vi "Down Pressure.vi"(5 "Direction":T1, 7 "init":bool, 8 "error in (no error)":errorcluster, 11 "Stand in":refnum<class "Stand.lvclass">) -> (0 "error out":errorcluster, 2 "done":bool, 3 "Stand out":refnum<class "Stand.lvclass">)   [LabVIEW 2019, in "Stand.lvclass"]
uses:
  Stand.lvclass
  TypeDef/Direction.ctl
  C:/Users/ANENKOV_V1/Desktop/src/Device_class/Device.lvclass
  TypeDef/State - Pressure Down.ctl
  Stand.lvclass/Stand.ctl
  AI_class/AI.lvclass/AI.ctl
  AnalogComparator_class/AnalogComparator.lvclass/AnalogComparator.ctl
  Device_class/Device.lvclass/Device.ctl
  FPGA/TypeDef/DO index.ctl
  NeedleValve_class/Cmd.ctl
  f8234472-8bf1-448c-8c25-8d9f60be58e1.vi
  AnalogComparator_class/GetStatus.vi
  FPGA_API_class/FPGA API.lvclass
  Device_class/Device.lvclass
  AI_class/AI.lvclass
  NeedleValve_class/NeedleValve.lvclass
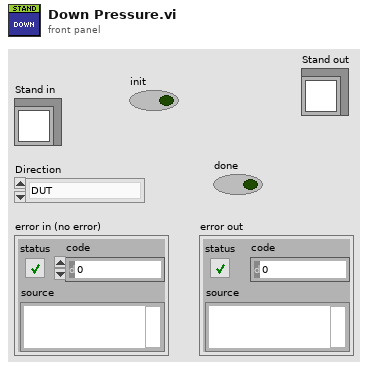
[diagram p1: front panel]
types:
  T1 = typedef "Direction.ctl" = enum8{"DUT", "Chamber"}
  T2 = typedef "State - Pressure Down.ctl" = enum16{"Check", "Close Inlet", "Open Outlet", "Down", "Exit"}
  T3 = typedef "NeedleValve.lvclass/Cmd.ctl" = enum16{"Open", "Close", "Stop"}
  T4 = typedef "AI_Data.ctl" = cluster{"Stat Data":T5, "OutOfRangeMax":bool, "OutOfRangeMin":bool, "HIHI":bool, "HI":bool, "LO":bool, "LOLO":bool}
  T5 = typedef "AI Statistics Data.ctl" = cluster{"raw mean":dbl, "scl mean":dbl, "raw mean 1Hz":dbl, "scl mean 1Hz":dbl}
  T6 = typedef "DO index.ctl" = u8
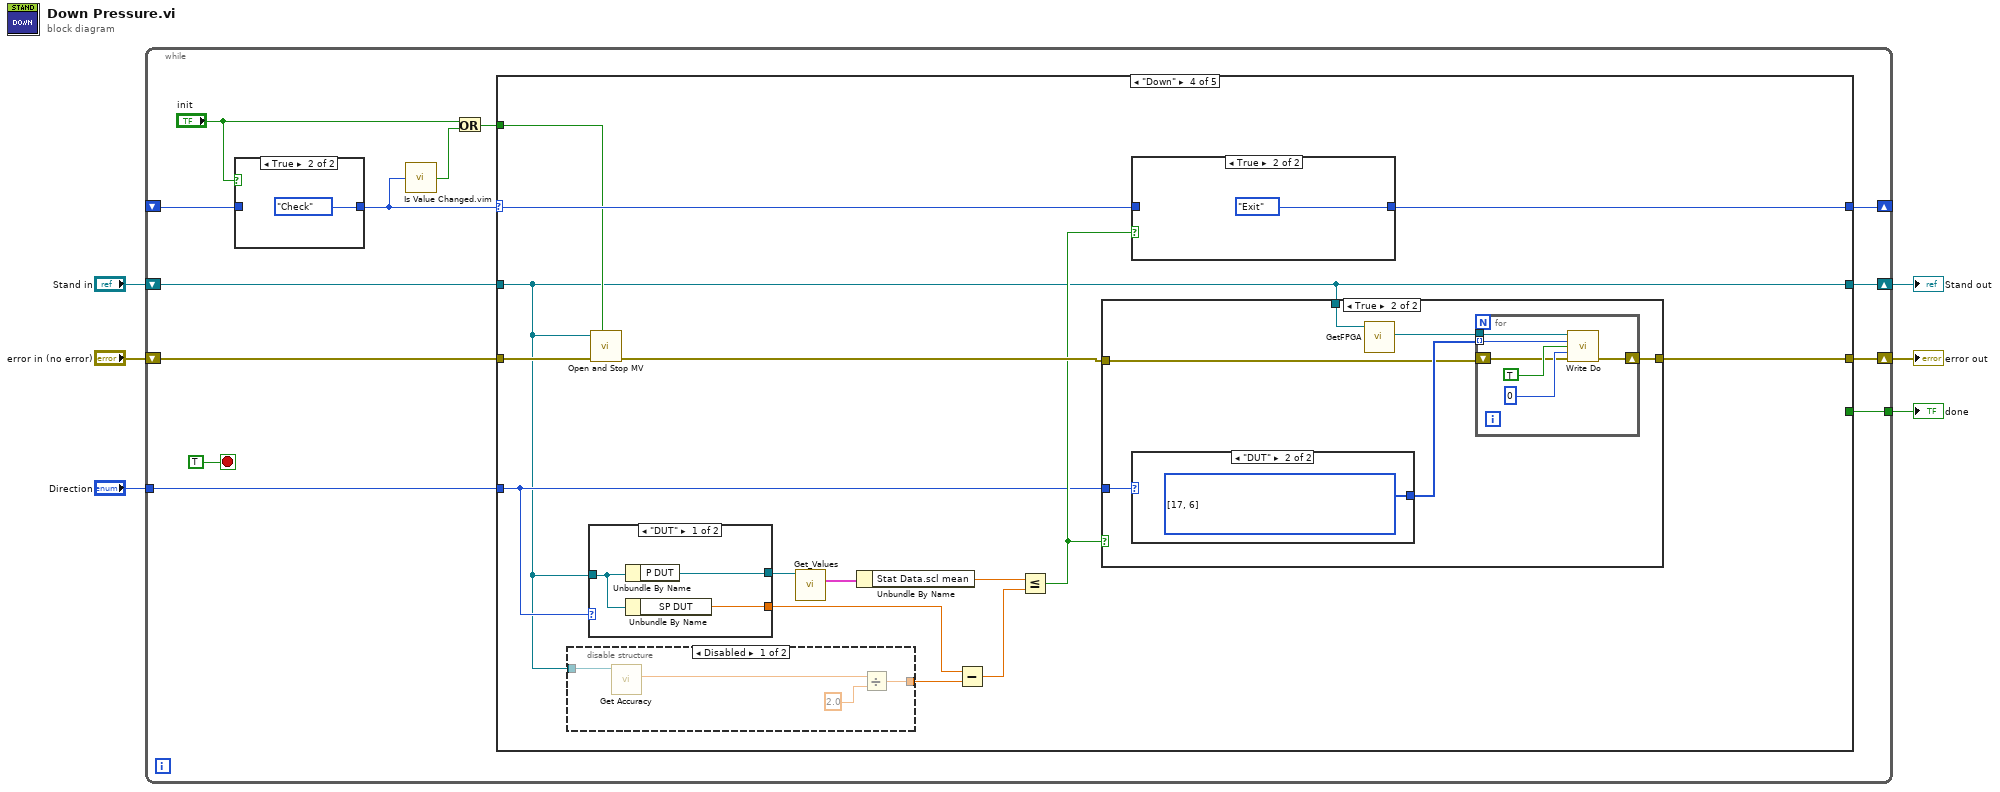
[diagram p0: block diagram]
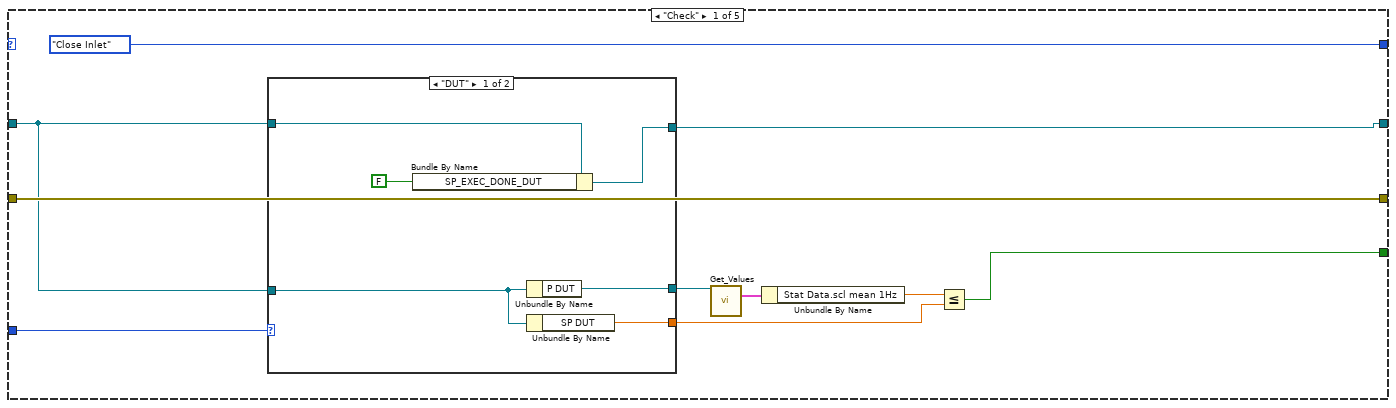
[diagram p2: hidden frame]
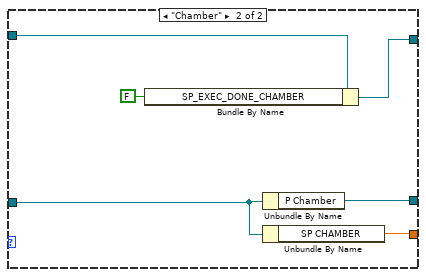
[diagram p3: hidden frame]
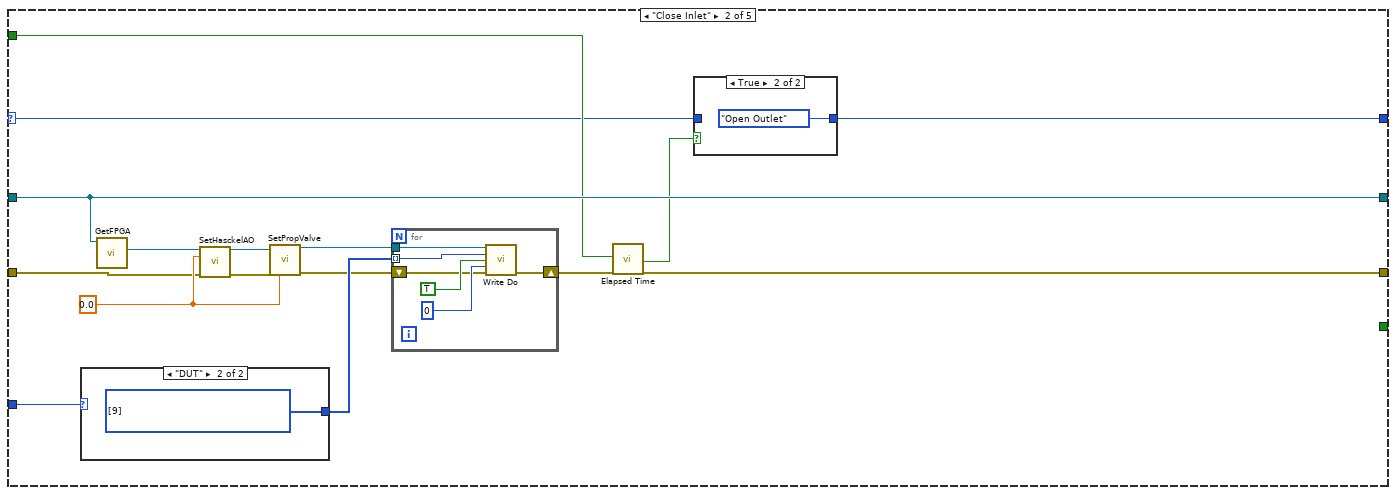
[diagram p4: hidden frame]
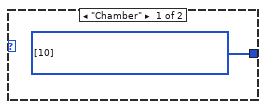
[diagram p6: hidden frame]
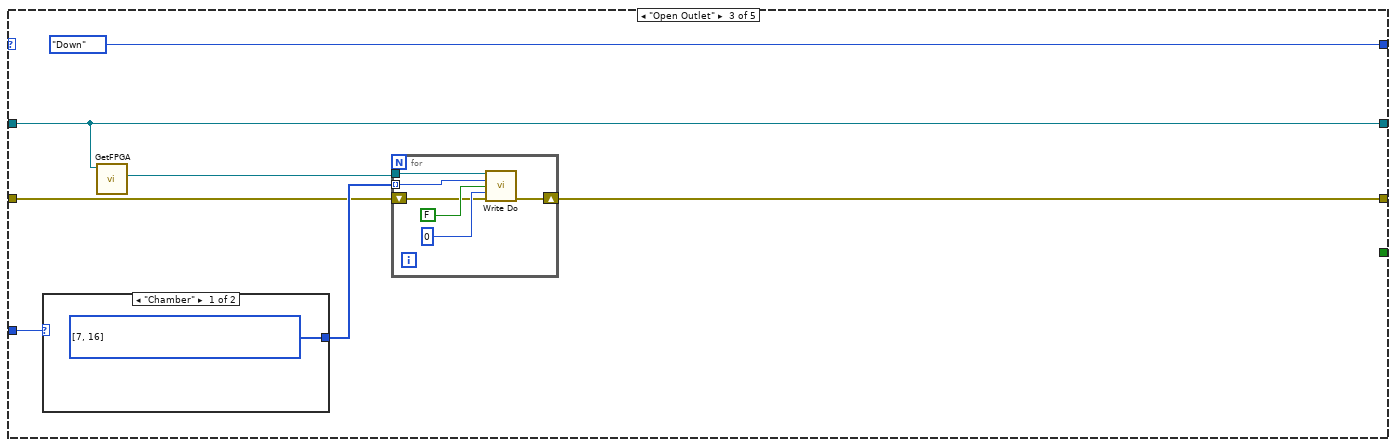
[diagram p7: hidden frame]
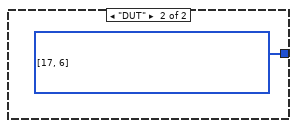
[diagram p8: hidden frame]
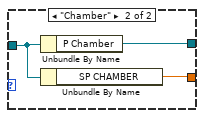
[diagram p10: hidden frame]
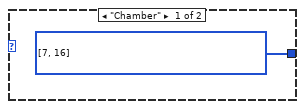
[diagram p13: hidden frame]
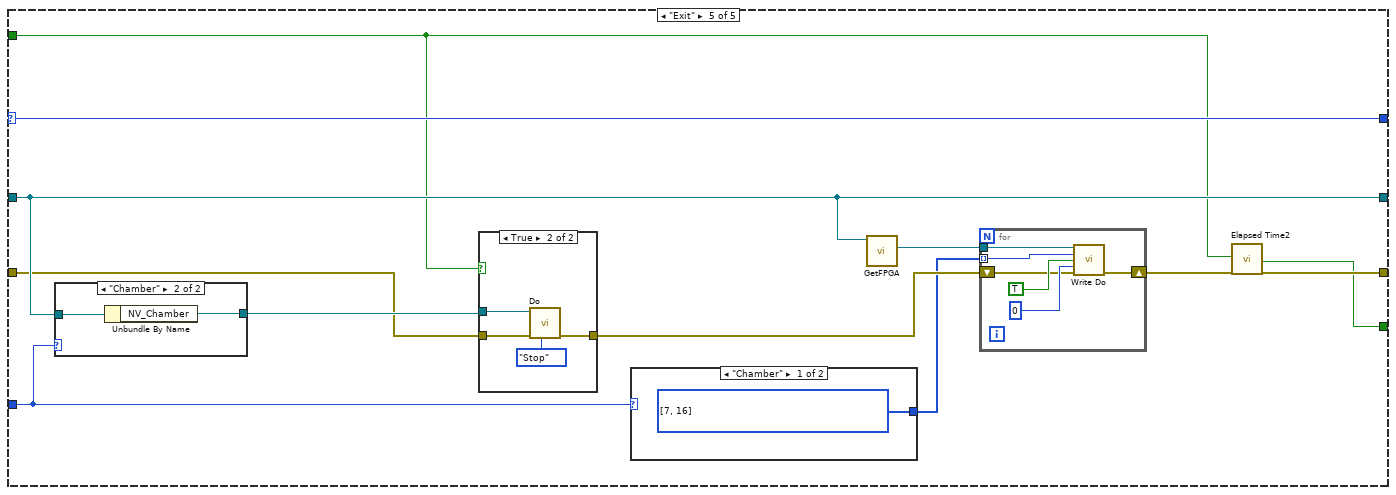
[diagram p14: hidden frame]
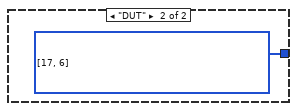
[diagram p15: hidden frame]
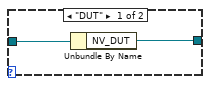
[diagram p17: hidden frame]
diagram:
  n1 = while {
    shift-right: [w11] -> w2
    shift-left: "error in (no error)" -> [w10]
    tunnel: "Direction" -> [w7]
    shift-right: [w12] -> w3
    shift-left: "Stand in" -> [w9]
    shift-right: [w18] -> _
    shift-left: _ -> [w17]
    tunnel: [w8] -> w1
    stop <- TRUE stop-if-true
    n2 = case shown="True" "init" {
      tunnel: [w154 State_-_Pressure_Down."Check"] -> w16
      tunnel: w17 -> [w154 _]
      frame False {
      }
      frame True {
      }
    }
    n3 = call "Is Value Changed.vim"("value"=w16) -> ("changed or first call?"=w14:bool)
    n4 = Or(x="init", y=w14) -> (x .or. y?=w13:bool)
    n5 = case shown="\"Down\"" w16 {
      selector: w16 -> [_ w44 _ w93 w133]
      tunnel: w9 -> [w21 w49 w71 w86 w135]
      tunnel: [State_-_Pressure_Down."Close Inlet" w45 State_-_Pressure_Down."Down" w94 w133] -> w18
      tunnel: w13 -> [_ w47 _ w87 w126]
      tunnel: [w20 w49 w71 w86 w135] -> w12
      tunnel: [w29 w43 w70 w97 w127] -> w11
      tunnel: w10 -> [w29 w50 w72 w95 w129]
      tunnel: w7 -> [w23 w42 w68 w88 w136]
      tunnel: [w22 _ _ _ w125] -> w8
      frame "Check" {
        n6 = case shown="\"DUT\"" w23 {
          tunnel: [w35 w41] -> w26
          tunnel: [w34 w40] -> w24
          tunnel: w21 -> [w33 w39]
          tunnel: w21 -> [w31 w38]
          tunnel: [w30 w37] -> w20
          frame "DUT" {
            n7 = Bundle By Name(cluster=w31, "SP_EXEC_DONE_DUT"=FALSE ("Data.STS.SP_EXEC_DONE_CHAMBER")) -> (w30:refnum<class "Stand.lvclass">)
            n8 = Unbundle By Name(w33) -> ("P DUT"=w35:refnum<class "AI.lvclass">)
            n9 = Unbundle By Name(w33) -> ("SP DUT"=w34:dbl)
          }
          frame "Chamber" {
            n10 = Bundle By Name(cluster=w38, "SP_EXEC_DONE_CHAMBER"=FALSE ("Data.STS.SP_EXEC_DONE_CHAMBER")) -> (w37:refnum<class "Stand.lvclass">)
            n11 = Unbundle By Name(w39) -> ("P Chamber"=w41:refnum<class "AI.lvclass">)
            n12 = Unbundle By Name(w39) -> ("SP CHAMBER"=w40:dbl)
          }
        }
        n13 = call "Get_Values.vi"("reference in"=w26) -> ("Data"=w27:T4)  [unwired: 14 in]
        n14 = Unbundle By Name(w27) -> ("Stat Data.scl mean 1Hz"=w25:dbl)
        n15 = Less Or Equal?(x=w25, y=w24) -> (x <= y?=w22:bool)
      }
      frame "Close Inlet" {
        w51 = 0.0 ("Haskel in")
        n16 = case shown="\"DUT\"" w42 {
          tunnel: [w66 w67] -> w57
          frame "Chamber" {
            w66 = T6[] [10] items=["DO 0 [KP1] [M12]", "DO 1 [ON KP2] [M21]", "DO 2 [ON KP3] [M24]", "DO 3 [WATER Y18.1 [DO3]]", "DO 4 [WATER Y18.2 [DO4]]", "DO 5 [KP6 Y29.1 33.7]", "DO 6 [KP7 Y29.2 33.8]", "DO 7 [KP8 Y29.3 33.9]", "DO 8 [KP9 Y29.4  33.12]", "DO 9 [KP10 Y29.5 33.1]", "DO 10 [KP11 Y29.6 33.2]", "DO 11 [KP12 Y29.7  33.13]", "DO 12 [KP13 Y29.8  33.11]", "DO 13 [KP14 Y29.9 33.10]", "DO 14 [KP15 Y29.10  33.6]", "DO 15 [KP16 Y29.11  33.5]", "DO 16 [KP17 Y29.12  33.4]", "DO 17 [KP18 Y29.13 33.3]", "DO 18 [AIR KP19]", "DO 19 [STEP DRIVE EN KP20]", "DO 20 [KP21 Y44.1 OPEN]", "DO 21 [ KP22 Y44.1 CLOSE]", "DO 22 [ KP23 Y44.2 OPEN]", "DO 23", "DO 24 [STEP DRIVE 1]", "DO 25 [STEP DRIVE 2]"]
          }
          frame "DUT" {
            w67 = T6[] [9] items=["DO 0 [KP1] [M12]", "DO 1 [ON KP2] [M21]", "DO 2 [ON KP3] [M24]", "DO 3 [WATER Y18.1 [DO3]]", "DO 4 [WATER Y18.2 [DO4]]", "DO 5 [KP6 Y29.1 33.7]", "DO 6 [KP7 Y29.2 33.8]", "DO 7 [KP8 Y29.3 33.9]", "DO 8 [KP9 Y29.4  33.12]", "DO 9 [KP10 Y29.5 33.1]", "DO 10 [KP11 Y29.6 33.2]", "DO 11 [KP12 Y29.7  33.13]", "DO 12 [KP13 Y29.8  33.11]", "DO 13 [KP14 Y29.9 33.10]", "DO 14 [KP15 Y29.10  33.6]", "DO 15 [KP16 Y29.11  33.5]", "DO 16 [KP17 Y29.12  33.4]", "DO 17 [KP18 Y29.13 33.3]", "DO 18 [AIR KP19]", "DO 19 [STEP DRIVE EN KP20]", "DO 20 [KP21 Y44.1 OPEN]", "DO 21 [ KP22 Y44.1 CLOSE]", "DO 22 [ KP23 Y44.2 OPEN]", "DO 23", "DO 24 [STEP DRIVE 1]", "DO 25 [STEP DRIVE 2]"]
          }
        }
        n17 = call "GetFPGA.vi"("Device in"=w49) -> ("FPGA API.lvclass"=w52:refnum<class "FPGA API.lvclass">)  [unwired: 10 in]
        n18 = call-dynamic "SetHasckelAO.vi"("FPGA API in"=w52, "Haskel in"=w51, "error in (no error)"=w50) -> ("FPGA API out"=w54:refnum<class "FPGA API.lvclass">, "error out"=w53:errorcluster)  [unwired: 11 in]
        n19 = call-dynamic "SetPropValve.vi"("FPGA API in"=w54, "error in (no error)"=w53, "AO 1"=w51) -> ("FPGA API out"=w55:refnum<class "FPGA API.lvclass">, "error out"=w56:errorcluster)  [unwired: 11 in]
        n20 = for {
          tunnel: w55 -> [w63]
          tunnel: w57 -> [w61] mode=indexing
          shift-right: [w60] -> w48
          shift-left: w56 -> [w62]
          n21 = call-dynamic "Write Do.vi"("FPGA API in"=w63, "#DO"=w61, "value"=TRUE, "Time uSec"=u32 0, "error in (no error)"=w62) -> ("error out"=w60:errorcluster)  [unwired: 9 in, 1 out]
        }
        n22 = call "Elapsed Time"("Reset"=w47, "error in (no error)"=w48) -> ("Time has Elapsed"=w46:bool, "error out"=w43:errorcluster)  [unwired: 10 in, 6 out]
        n23 = case shown="True" w46 {
          tunnel: [w58 State_-_Pressure_Down."Open Outlet"] -> w45
          tunnel: w44 -> [w58 _]
          frame False {
          }
          frame True {
          }
        }
      }
      frame "Open Outlet" {
        n24 = case shown="\"Chamber\"" w68 {
          tunnel: [w81 w82] -> w74
          frame "Chamber" {
            w81 = T6[] [7, 16] items=["DO 0 [KP1] [M12]", "DO 1 [ON KP2] [M21]", "DO 2 [ON KP3] [M24]", "DO 3 [WATER Y18.1 [DO3]]", "DO 4 [WATER Y18.2 [DO4]]", "DO 5 [KP6 Y29.1 33.7]", "DO 6 [KP7 Y29.2 33.8]", "DO 7 [KP8 Y29.3 33.9]", "DO 8 [KP9 Y29.4  33.12]", "DO 9 [KP10 Y29.5 33.1]", "DO 10 [KP11 Y29.6 33.2]", "DO 11 [KP12 Y29.7  33.13]", "DO 12 [KP13 Y29.8  33.11]", "DO 13 [KP14 Y29.9 33.10]", "DO 14 [KP15 Y29.10  33.6]", "DO 15 [KP16 Y29.11  33.5]", "DO 16 [KP17 Y29.12  33.4]", "DO 17 [KP18 Y29.13 33.3]", "DO 18 [AIR KP19]", "DO 19 [STEP DRIVE EN KP20]", "DO 20 [KP21 Y44.1 OPEN]", "DO 21 [ KP22 Y44.1 CLOSE]", "DO 22 [ KP23 Y44.2 OPEN]", "DO 23", "DO 24 [STEP DRIVE 1]", "DO 25 [STEP DRIVE 2]"]
          }
          frame "DUT" {
            w82 = T6[] [17, 6] items=["DO 0 [KP1] [M12]", "DO 1 [ON KP2] [M21]", "DO 2 [ON KP3] [M24]", "DO 3 [WATER Y18.1 [DO3]]", "DO 4 [WATER Y18.2 [DO4]]", "DO 5 [KP6 Y29.1 33.7]", "DO 6 [KP7 Y29.2 33.8]", "DO 7 [KP8 Y29.3 33.9]", "DO 8 [KP9 Y29.4  33.12]", "DO 9 [KP10 Y29.5 33.1]", "DO 10 [KP11 Y29.6 33.2]", "DO 11 [KP12 Y29.7  33.13]", "DO 12 [KP13 Y29.8  33.11]", "DO 13 [KP14 Y29.9 33.10]", "DO 14 [KP15 Y29.10  33.6]", "DO 15 [KP16 Y29.11  33.5]", "DO 16 [KP17 Y29.12  33.4]", "DO 17 [KP18 Y29.13 33.3]", "DO 18 [AIR KP19]", "DO 19 [STEP DRIVE EN KP20]", "DO 20 [KP21 Y44.1 OPEN]", "DO 21 [ KP22 Y44.1 CLOSE]", "DO 22 [ KP23 Y44.2 OPEN]", "DO 23", "DO 24 [STEP DRIVE 1]", "DO 25 [STEP DRIVE 2]"]
          }
        }
        n25 = call "GetFPGA.vi"("Device in"=w71) -> ("FPGA API.lvclass"=w73:refnum<class "FPGA API.lvclass">)  [unwired: 10 in]
        n26 = for {
          tunnel: w73 -> [w78]
          tunnel: w74 -> [w76] mode=indexing
          shift-right: [w75] -> w70
          shift-left: w72 -> [w77]
          n27 = call-dynamic "Write Do.vi"("FPGA API in"=w78, "#DO"=w76, "value"=FALSE, "Time uSec"=u32 0, "error in (no error)"=w77) -> ("error out"=w75:errorcluster)  [unwired: 9 in, 1 out]
        }
      }
      frame "Down" {
        n28 = disable-structure shown="Disabled" {
          disable-tunnel: w86 -> [w100 _]
          disable-tunnel: [w98 _] -> w85
          frame Disabled {
            n29 = call "Get Accuracy.vi"("Stand in"=w100) -> ("Accuracy [MPa]"=w99:dbl)  [unwired: 10 in]
            n30 = Divide(x=w99, y=2.0) -> (x/y=w98:dbl)
          }
          frame Enabled {
          }
        }
        n31 = case shown="\"DUT\"" w88 {
          tunnel: [w104 w107] -> w91
          tunnel: [w103 w106] -> w84
          tunnel: w86 -> [w102 w105]
          frame "DUT" {
            n32 = Unbundle By Name(w102) -> ("P DUT"=w104:refnum<class "AI.lvclass">)
            n33 = Unbundle By Name(w102) -> ("SP DUT"=w103:dbl)
          }
          frame "Chamber" {
            n34 = Unbundle By Name(w105) -> ("P Chamber"=w107:refnum<class "AI.lvclass">)
            n35 = Unbundle By Name(w105) -> ("SP CHAMBER"=w106:dbl)
          }
        }
        n36 = call "Open and Stop MV.vi"("init"=w87, "error in (no error)"=w95, "Stand in"=w86) -> ("error out"=w96:errorcluster)  [unwired: 8 in]
        n37 = call "Get_Values.vi"("reference in"=w91) -> ("Data"=w92:T4)  [unwired: 14 in]
        n38 = Unbundle By Name(w92) -> ("Stat Data.scl mean"=w90:dbl)
        n39 = Subtract(x=w84, y=w85) -> (x-y=w83:dbl)
        n40 = Less Or Equal?(x=w90, y=w83) -> (x <= y?=w89:bool)
        n41 = case shown="True" w89 {
          tunnel: w88 -> [_ w114]
          tunnel: [w110 w113] -> w97
          tunnel: w86 -> [_ w112]
          tunnel: w96 -> [w110 w111]
          frame False {
          }
          frame True {
            n42 = case shown="\"DUT\"" w114 {
              tunnel: [w123 w124] -> w116
              frame "Chamber" {
                w123 = T6[] [7, 16] items=["DO 0 [KP1] [M12]", "DO 1 [ON KP2] [M21]", "DO 2 [ON KP3] [M24]", "DO 3 [WATER Y18.1 [DO3]]", "DO 4 [WATER Y18.2 [DO4]]", "DO 5 [KP6 Y29.1 33.7]", "DO 6 [KP7 Y29.2 33.8]", "DO 7 [KP8 Y29.3 33.9]", "DO 8 [KP9 Y29.4  33.12]", "DO 9 [KP10 Y29.5 33.1]", "DO 10 [KP11 Y29.6 33.2]", "DO 11 [KP12 Y29.7  33.13]", "DO 12 [KP13 Y29.8  33.11]", "DO 13 [KP14 Y29.9 33.10]", "DO 14 [KP15 Y29.10  33.6]", "DO 15 [KP16 Y29.11  33.5]", "DO 16 [KP17 Y29.12  33.4]", "DO 17 [KP18 Y29.13 33.3]", "DO 18 [AIR KP19]", "DO 19 [STEP DRIVE EN KP20]", "DO 20 [KP21 Y44.1 OPEN]", "DO 21 [ KP22 Y44.1 CLOSE]", "DO 22 [ KP23 Y44.2 OPEN]", "DO 23", "DO 24 [STEP DRIVE 1]", "DO 25 [STEP DRIVE 2]"]
              }
              frame "DUT" {
                w124 = T6[] [17, 6] items=["DO 0 [KP1] [M12]", "DO 1 [ON KP2] [M21]", "DO 2 [ON KP3] [M24]", "DO 3 [WATER Y18.1 [DO3]]", "DO 4 [WATER Y18.2 [DO4]]", "DO 5 [KP6 Y29.1 33.7]", "DO 6 [KP7 Y29.2 33.8]", "DO 7 [KP8 Y29.3 33.9]", "DO 8 [KP9 Y29.4  33.12]", "DO 9 [KP10 Y29.5 33.1]", "DO 10 [KP11 Y29.6 33.2]", "DO 11 [KP12 Y29.7  33.13]", "DO 12 [KP13 Y29.8  33.11]", "DO 13 [KP14 Y29.9 33.10]", "DO 14 [KP15 Y29.10  33.6]", "DO 15 [KP16 Y29.11  33.5]", "DO 16 [KP17 Y29.12  33.4]", "DO 17 [KP18 Y29.13 33.3]", "DO 18 [AIR KP19]", "DO 19 [STEP DRIVE EN KP20]", "DO 20 [KP21 Y44.1 OPEN]", "DO 21 [ KP22 Y44.1 CLOSE]", "DO 22 [ KP23 Y44.2 OPEN]", "DO 23", "DO 24 [STEP DRIVE 1]", "DO 25 [STEP DRIVE 2]"]
              }
            }
            n43 = call "GetFPGA.vi"("Device in"=w112) -> ("FPGA API.lvclass"=w115:refnum<class "FPGA API.lvclass">)  [unwired: 10 in]
            n44 = for {
              tunnel: w115 -> [w120]
              tunnel: w116 -> [w118] mode=indexing
              shift-right: [w117] -> w113
              shift-left: w111 -> [w119]
              n45 = call-dynamic "Write Do.vi"("FPGA API in"=w120, "#DO"=w118, "value"=TRUE, "Time uSec"=u32 0, "error in (no error)"=w119) -> ("error out"=w117:errorcluster)  [unwired: 9 in, 1 out]
            }
          }
        }
        n46 = case shown="True" w89 {
          tunnel: [w108 State_-_Pressure_Down."Exit"] -> w94
          tunnel: w93 -> [w108 _]
          frame False {
          }
          frame True {
          }
        }
      }
      frame "Exit" {
        n47 = case shown="\"Chamber\"" w136 {
          tunnel: [w151 w153] -> w130
          tunnel: w135 -> [w150 w152]
          frame "DUT" {
            n48 = Unbundle By Name(w150) -> ("NV_DUT"=w151:refnum<class "NeedleValve.lvclass">)
          }
          frame "Chamber" {
            n49 = Unbundle By Name(w152) -> ("NV_Chamber"=w153:refnum<class "NeedleValve.lvclass">)
          }
        }
        n50 = case shown="True" w126 {
          tunnel: [w145 w149] -> w134
          tunnel: w130 -> [_ w147]
          tunnel: w129 -> [w145 w146]
          frame False {
          }
          frame True {
            n51 = call "Do.vi"("Cmd"=Cmd."Stop", "error in (no error)"=w146, "NeedleValve in"=w147) -> ("error out"=w149:errorcluster)  [unwired: 7 in, 1 out]
          }
        }
        n52 = case shown="\"Chamber\"" w136 {
          tunnel: [w143 w144] -> w132
          frame "Chamber" {
            w143 = T6[] [7, 16] items=["DO 0 [KP1] [M12]", "DO 1 [ON KP2] [M21]", "DO 2 [ON KP3] [M24]", "DO 3 [WATER Y18.1 [DO3]]", "DO 4 [WATER Y18.2 [DO4]]", "DO 5 [KP6 Y29.1 33.7]", "DO 6 [KP7 Y29.2 33.8]", "DO 7 [KP8 Y29.3 33.9]", "DO 8 [KP9 Y29.4  33.12]", "DO 9 [KP10 Y29.5 33.1]", "DO 10 [KP11 Y29.6 33.2]", "DO 11 [KP12 Y29.7  33.13]", "DO 12 [KP13 Y29.8  33.11]", "DO 13 [KP14 Y29.9 33.10]", "DO 14 [KP15 Y29.10  33.6]", "DO 15 [KP16 Y29.11  33.5]", "DO 16 [KP17 Y29.12  33.4]", "DO 17 [KP18 Y29.13 33.3]", "DO 18 [AIR KP19]", "DO 19 [STEP DRIVE EN KP20]", "DO 20 [KP21 Y44.1 OPEN]", "DO 21 [ KP22 Y44.1 CLOSE]", "DO 22 [ KP23 Y44.2 OPEN]", "DO 23", "DO 24 [STEP DRIVE 1]", "DO 25 [STEP DRIVE 2]"]
          }
          frame "DUT" {
            w144 = T6[] [17, 6] items=["DO 0 [KP1] [M12]", "DO 1 [ON KP2] [M21]", "DO 2 [ON KP3] [M24]", "DO 3 [WATER Y18.1 [DO3]]", "DO 4 [WATER Y18.2 [DO4]]", "DO 5 [KP6 Y29.1 33.7]", "DO 6 [KP7 Y29.2 33.8]", "DO 7 [KP8 Y29.3 33.9]", "DO 8 [KP9 Y29.4  33.12]", "DO 9 [KP10 Y29.5 33.1]", "DO 10 [KP11 Y29.6 33.2]", "DO 11 [KP12 Y29.7  33.13]", "DO 12 [KP13 Y29.8  33.11]", "DO 13 [KP14 Y29.9 33.10]", "DO 14 [KP15 Y29.10  33.6]", "DO 15 [KP16 Y29.11  33.5]", "DO 16 [KP17 Y29.12  33.4]", "DO 17 [KP18 Y29.13 33.3]", "DO 18 [AIR KP19]", "DO 19 [STEP DRIVE EN KP20]", "DO 20 [KP21 Y44.1 OPEN]", "DO 21 [ KP22 Y44.1 CLOSE]", "DO 22 [ KP23 Y44.2 OPEN]", "DO 23", "DO 24 [STEP DRIVE 1]", "DO 25 [STEP DRIVE 2]"]
          }
        }
        n53 = call "GetFPGA.vi"("Device in"=w135) -> ("FPGA API.lvclass"=w131:refnum<class "FPGA API.lvclass">)  [unwired: 10 in]
        n54 = for {
          tunnel: w131 -> [w140]
          tunnel: w132 -> [w138] mode=indexing
          shift-right: [w137] -> w128
          shift-left: w134 -> [w139]
          n55 = call-dynamic "Write Do.vi"("FPGA API in"=w140, "#DO"=w138, "value"=TRUE, "Time uSec"=u32 0, "error in (no error)"=w139) -> ("error out"=w137:errorcluster)  [unwired: 9 in, 1 out]
        }
        n56 = call "Elapsed Time2"("Reset"=w126, "error in (no error)"=w128) -> ("Time has Elapsed"=w125:bool, "error out"=w127:errorcluster)  [unwired: 10 in, 6 out]
      }
    }
  }
  "error out" <- w2
  "Stand out" <- w3
  "done" <- w1
